vi "INFO.VER FPGA.vi"(7 "Espera acceso FT":u32, 8 "error out 2":errorcluster, 11 "FT_Handle":u32) -> (0 "error out":errorcluster, 2 "Numeric":u8, 3 "ftHandle_out":u32)   [LabVIEW 2019]
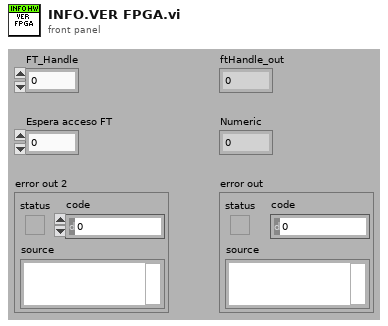
[diagram p1: front panel]
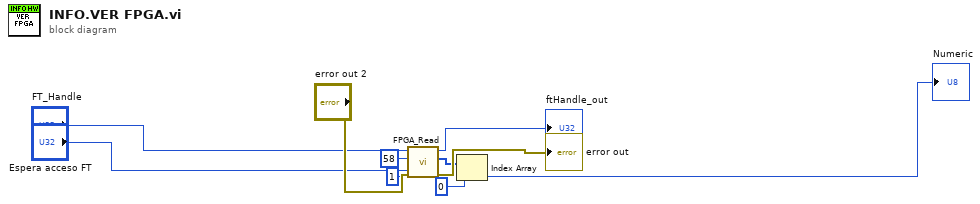
[diagram p0: block diagram]
diagram:
  n1 = call "FPGA_Read.vi"("Espera acceso USB"="Espera acceso FT", "error in"="error out 2", "Numero Bytes"=u8 1, "Dirección base"=u8 58, "ftHandle_in"="FT_Handle") -> ("error out"=→"error out":errorcluster, "lpBuffer_out"=w5:u8[], "ftHandle_out"=→"ftHandle_out":u32)  [unwired: 2 in, 2 out]
  n2 = Index Array(array=w5, index=0) -> (element=→"Numeric":u8)
